vi "NortekInstruction.vi"() -> ()   [LabVIEW 2015]
panel:
  in  "CommandeNortek":string
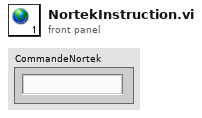
[diagram p1: front panel]
diagram:
